vi "FPGA Main R3 AB JC KV.vi"() -> ()   [LabVIEW 2018]
uses:
  Type Defs/Control Mode.ctl
  <vilib>/rvi/Emulation/niFpgaGetClockAttributes.vi
  <vilib>/rvi/Emulation/niFpgaSctlEmulationGetInTimedLoop.vi
  <vilib>/rvi/Emulation/niFpgaEmulationReportErrorSimple.vi
  <vilib>/rvi/eio/common/nirviEmuTemplateMethod_errors.vi
  <vilib>/rvi/Emulation/niFpgaProcessEmulError.vi
  <vilib>/rvi/interface/RandomDataEmulation/niFpgaRandomDataHandleErrors.vi
  <vilib>/rvi/Emulation/niFpgaCriticalErrorInLSC.vi
  <vilib>/rvi/Analysis/control/PID/SubVIs/niFpgaPID_PIWrapper.vi
  <vilib>/eio/EIONode/EIONode.xnode
  <vilib>/rvi/DataTransferAndStorage/Container/XNode/niFpgaContainer.xnode
  <vilib>/rvi/interface/RandomDataEmulation/nirviRandomDataFpgaReadWriteTemplate.vi
panel:
  out "Measuring?":bool
  in  "FIFO":bool
  in  "FFWD/PID":bool
  in  "Amplifier On/Off":bool
  out "Current Mode":T1
  out "Array Index":i32
  in  "Control Mode":T1
  out "PID Error (V)":sgl
  out "PID Output (V)":u16
  in  "Output Limits":cluster{"Vmax":sgl, "Vmin":sgl}
  in  "PID Gains":cluster{"Kp":sgl, "Ki":sgl}
  out "Capacitance\nProbe (V)":u16
  out "Coil Back \nEMF (V)":u16
  in  "Control Loop \nRate (uSec)":u32
  in  "Sensor Loop \nRate (uSec)":u32
  in  "VC Command (V)":u16
  # "Sensors"
  # "Loop Rates"
  # "Controls"
  # "PID Settings"
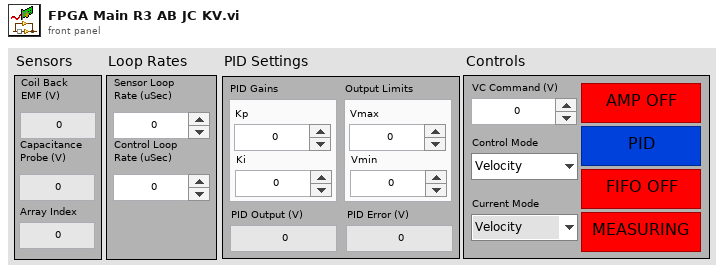
[diagram p1: front panel]
types:
  T1 = typedef "Control Mode.ctl" = enum16{"Velocity", "Displacement", "Manual", "Load Sine"}
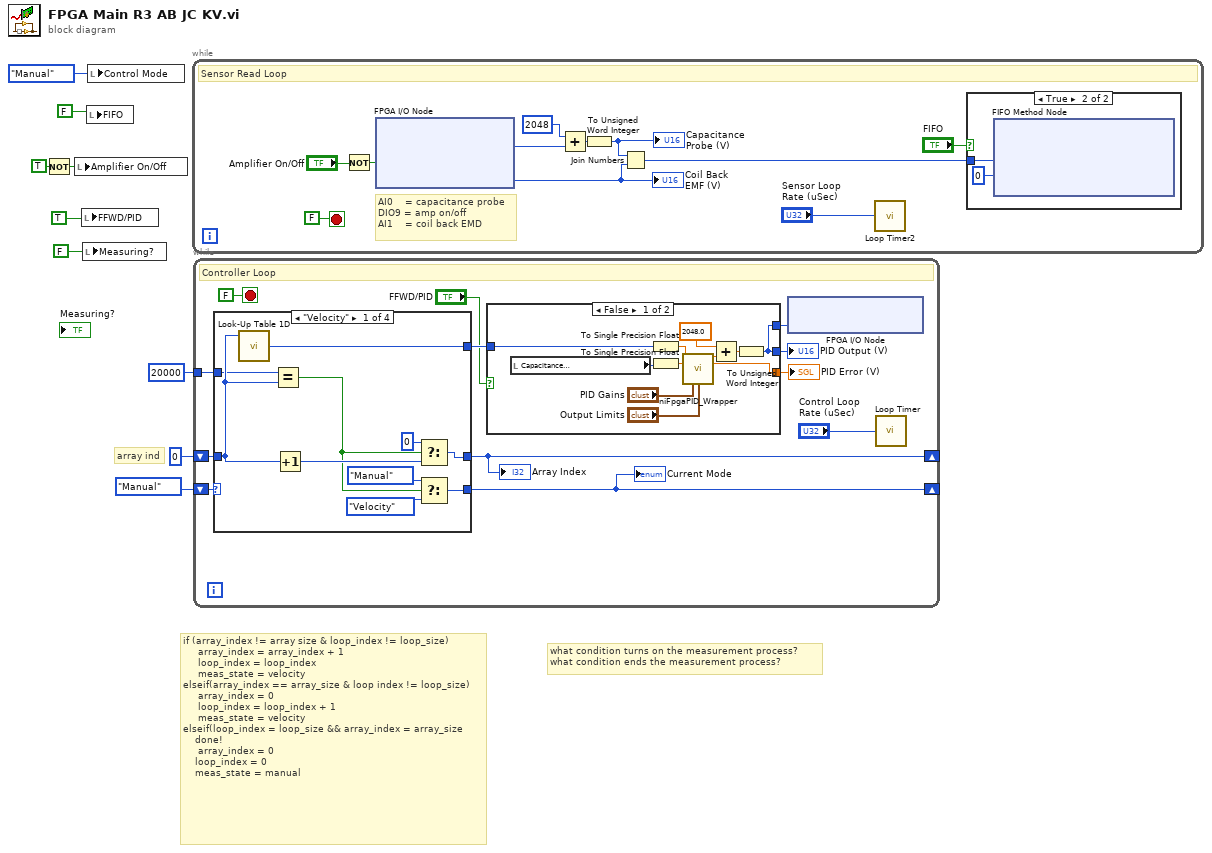
[diagram p0: block diagram]
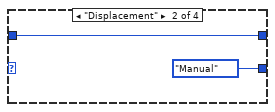
[diagram p2: hidden frame]
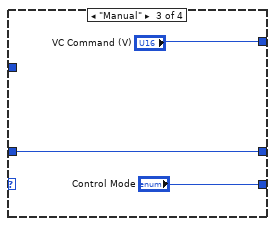
[diagram p3: hidden frame]
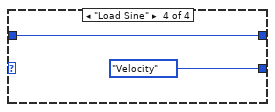
[diagram p4: hidden frame]
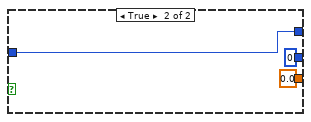
[diagram p5: hidden frame]
diagram:
  # "what condition turns on the measurement process?\nwhat condition ends the measurement process?"
  # "if (array_index != array size & loop_index != loop_size)\n     array_index = array_index + 1\n     loop_index = loop_index\n     meas_state = velocity\nelseif(array_index == array_size & loop index != loop_size)\n     array_index = 0\n     loop_index = loop_index + 1\n     meas_state = velocity\nelseif(loop_index = loop_size && array_index = array_size\n    done!\n     array_index = 0\n    loop_index = 0\n    meas_state = manual"
  # "array ind"
  n1 = Not(x=TRUE) -> (.not. x?=w5:bool)
  n2 = local write "Amplifier On/Off"(w5) -> ()
  n3 = local write "FFWD/PID"(TRUE) -> ()
  n4 = local write "Measuring?"(FALSE) -> ()
  n5 = local write "FIFO"(FALSE) -> ()
  n6 = local write "Control Mode"(Control_Mode."Manual" ("Control Mode")) -> ()
  n7 = while {
    stop <- FALSE stop-if-true
    # "AI0    = capacitance probe\nDIO9 = amp on/off\nAI1    = coil back EMD"
    # "Sensor Read Loop"
    n8 = Not(x="Amplifier On/Off") -> (.not. x?=w11:bool)
    n9 = xnode "FPGA I/O Node"("ConnectorA/DIO9"=w11) -> ("ConnectorC/AI0"=w19:i16, "ConnectorA/AI1"=w15:u16)  [unwired: 3 in, 3 out]
    "Coil Back \nEMF (V)" <- w15
    n10 = Add(x=i16 2048, y=w19) -> (x+y=w20:i16)
    n11 = To Unsigned Word Integer(number=w20) -> (unsigned 16bit integer=w14:u16)
    "Capacitance\nProbe (V)" <- w14
    n12 = Join Numbers(hi=w14, lo=w15) -> ((hi.lo)=w16:u32)
    n13 = call "Loop Timer2"("Count(uSec)"="Sensor Loop \nRate (uSec)") -> ()  [unwired: 1 out]
    n14 = case shown="True" "FIFO" {
      tunnel: w16 -> [_ w22]
      frame False {
      }
      frame True {
        n15 = xnode ("FIFO Method Node")("Element"=w22, "Timeout"=0) -> ()  [unwired: 1 in, 2 out]
      }
    }
  }
  n16 = while {
    shift-right: [w26] -> _
    shift-left: 0 ("index") -> [w29]
    shift-right: [w27] -> _
    shift-left: Control_Mode."Manual" ("Control Mode") -> [w28]
    tunnel: 20000 ("index") -> [w24]
    stop <- FALSE stop-if-true
    # "Controller Loop"
    n17 = case shown="\"Velocity\"" w28 {
      tunnel: [w36 _ "VC Command (V)" _] -> w33
      tunnel: w29 -> [w37 w45 w47 w51]
      tunnel: [w40 w45 w47 w51] -> w26
      tunnel: [w42 Control_Mode."Manual" ("Control Mode") "Control Mode" Control_Mode."Velocity" ("Control Mode")] -> w27
      tunnel: w24 -> [w35 _ _ _]
      frame "Velocity" {
        n18 = call "Look-Up Table 1D"("address"=w37) -> ("data out"=w36:u16)  [unwired: 8 in]
        n19 = Equal?(x=w35, y=w37) -> (x = y?=w38:bool)
        n20 = Increment(x=w37) -> (x+1=w41:i32)
        n21 = Select(t=0 ("index"), s=w38, f=w41) -> (s? t:f=w40:i32)
        n22 = Select(t=Control_Mode."Manual" ("Control Mode"), s=w38, f=Control_Mode."Velocity" ("Control Mode")) -> (s? t:f=w42:T1)
      }
      frame "Displacement" {
      }
      frame "Manual" {
      }
      frame "Load Sine" {
      }
    }
    "Current Mode" <- w27
    "Array Index" <- w26
    n23 = case shown="False" "FFWD/PID" {
      tunnel: w33 -> [w61 w63]
      tunnel: [w52 u16 0] -> w32
      tunnel: [w55 sgl 0.0 ("error")] -> w31
      tunnel: [w52 w63] -> w23
      frame False {
        n24 = local read "Capacitance\nProbe (V)"() -> (w59:u16)
        n25 = To Single Precision Float(number=w61) -> (single precision float=w60:sgl)
        n26 = To Single Precision Float(number=w59) -> (single precision float=w62:sgl)
        n27 = call-poly <vilib>:"niFpgaPID_Wrapper.vi"("setpoint"=w60, "process variable"=w62, "gains"="PID Gains", "output range"="Output Limits") -> ("output"=w54:sgl, "error"=w55:sgl)  [unwired: 9 in, 1 out]
        n28 = Add(x=sgl 2048.0, y=w54) -> (x+y=w56:sgl)
        n29 = To Unsigned Word Integer(number=w56) -> (unsigned 16bit integer=w52:u16)
      }
      frame True {
      }
    }
    "PID Output (V)" <- w32
    "PID Error (V)" <- w31
    n30 = xnode "FPGA I/O Node"("ConnectorA/AO1"=w23) -> ()  [unwired: 1 in, 1 out]
    n31 = call "Loop Timer"("Count(uSec)"="Control Loop \nRate (uSec)") -> ()  [unwired: 1 out]
  }
